vi "Read.vi"(8 "error in (no error)":errorcluster, 11 "ArduinoAIReal in":refnum<class "Arduino.lvclass">) -> (0 "error out":errorcluster, 2 "Response":string="519 \t519 \t518 \t518 \t518 \t518 \t518 \t519 \t518 \t518\t1023 \t1023 \t1023 \t1023 \t1023 \t1023 \t1023 \t1023 \t1023 \t1023\t45 \t45 \t45 \t45 \t46 \t45 \t46 \t45 \t46 \t46\t63 \t63 \t63 \t62 \t63 \t63 \t62 \t63 \t62 \t63\t0 \t1 \t0 \t1 \t0 \t1 \t0 \t0 \t1 \t1\t0 \t0 \t1 \t0 \t1 \t1 \t1 \t0 \t1 \t0\t\r\n", 3 "ArduinoAIReal out":refnum<class "Arduino.lvclass">)   [LabVIEW 2020, in "Arduino.lvlib" / "Arduino.lvclass"]
uses:
  Arduino.lvclass
  Arduino.lvclass/Arduino.ctl
panel:
  out "Number of Bytes at Serial Port":u32=246
  out "length":i32=246
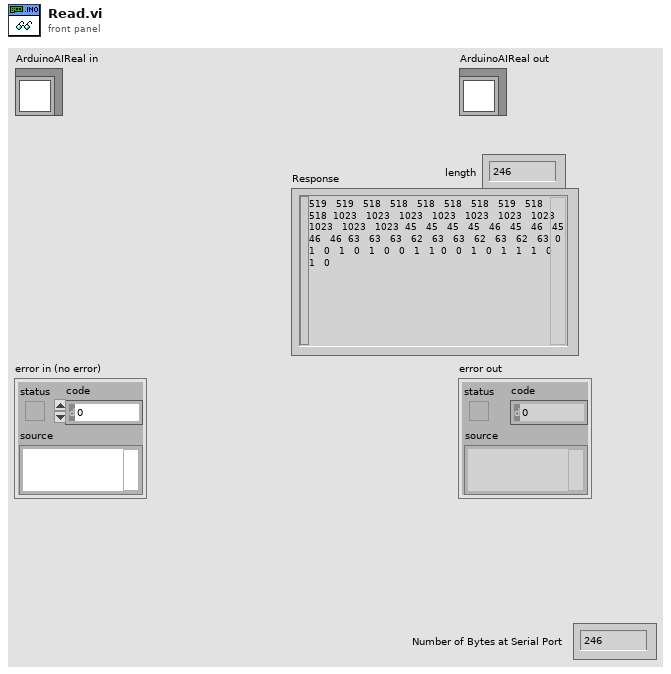
[diagram p1: front panel]
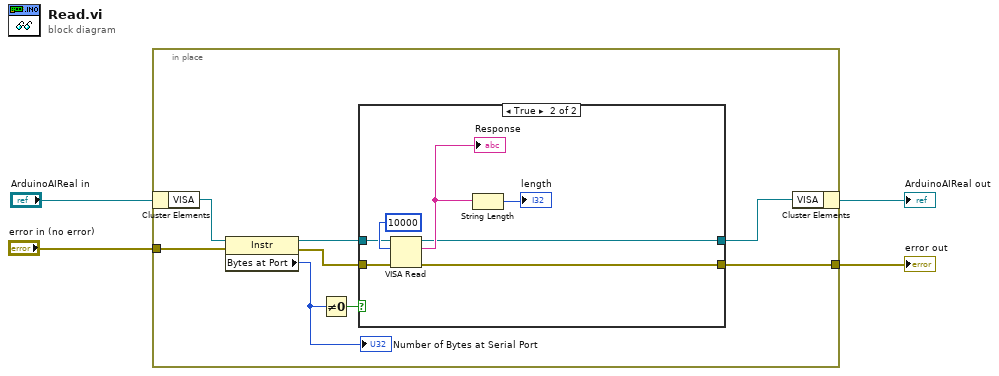
[diagram p0: block diagram]
diagram:
  n1 = in-place {
    in-place-border: "error in (no error)" -> [w8]
    in-place-border: [w7] -> w3
    n2 = in-place-cluster #1("ArduinoAIReal in") -> ("VISA"=w6:refnum<visa-resource-name>)
    n3 = property class="Instr"(reference=w6, error in=w8) -> (reference out=w12:refnum<visa-resource-name>, error out=w9:errorcluster, "Bytes at Port"=w11:u32)
    "Number of Bytes at Serial Port" <- w11
    n4 = Not Equal To 0?(x=w11) -> (x != 0?=w10:bool)
    n5 = case shown="True" w10 {
      tunnel: [w14 w16] -> w5
      tunnel: w9 -> [w13 w21]
      tunnel: [w13 w15] -> w7
      tunnel: w12 -> [w14 w19]
      frame False {
      }
      frame True {
        n6 = VISA Read(VISA resource name=w19, byte count=u32 10000 ("Read Count"), error in (no error)=w21) -> (VISA resource name out=w16:refnum<visa-resource-name>, read buffer=w18:string, error out=w15:errorcluster)  [unwired: 1 out]
        "Response" <- w18
        n7 = String Length(string=w18) -> (length=→"length":i32)
      }
    }
    n8 = in-place-cluster #1("VISA"=w5) -> (→"ArduinoAIReal out":refnum<class "Arduino.lvclass">)
  }
  "error out" <- w3
